vi "test_EnumerateServicesWrapper_RunEnumerateServices_ReturnsAvailableServices.vi"(8 "error in":errorcluster) -> (0 "error out":errorcluster, 2 "result":string, 3 "pass":bool)   [LabVIEW 2021, in "MeasurementServerTests.lvlib" / "Discovery Tests.lvlib"]
uses:
  Discovery Tests.lvlib
  MeasurementServerTests.lvlib
  gRPC/Generated APIs/ni/measurementlink/discovery/v1/RPC Messages/ni_measurementlink_discovery_v1_EnumerateServicesRequest.ctl
  gRPC/Generated APIs/ni/measurementlink/discovery/v1/ni.measurementlink.discovery.v1.api.lvlib
  Runtime/Clients/Discovery V1/NI Discovery V1 Client.lvlib
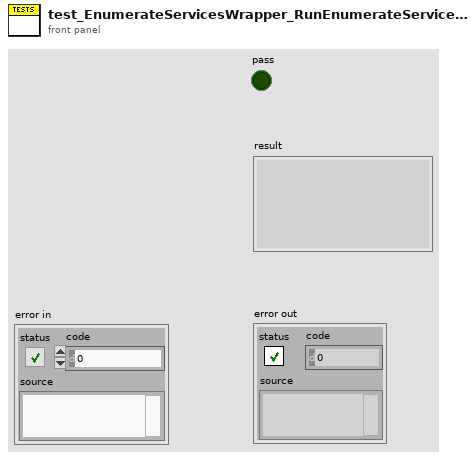
[diagram p1: front panel]
types:
  T1 = typedef "ni.measurementlink.discovery.v1.api.lvlib/ni_measurementlink_discovery_v1_EnumerateServicesRequest.ctl" = cluster{"provided_interface":string}
  T2 = typedef "ni.measurementlink.discovery.v1.api.lvlib/ni_measurementlink_discovery_v1_EnumerateServicesResponse.ctl" = cluster{"available_services":T3[]}
  T3 = typedef "ni.measurementlink.discovery.v1.api.lvlib/ni_measurementlink_discovery_v1_ServiceDescriptor.ctl" = cluster{"display_name":string, "description_url":string, "provided_interfaces":string[], "service_class":string, "annotations":T4[]}
  T4 = typedef "ni.measurementlink.discovery.v1.api.lvlib/ni_measurementlink_discovery_v1_ServiceDescriptor_AnnotationsEntry.ctl" = cluster{"key":string, "value":string}
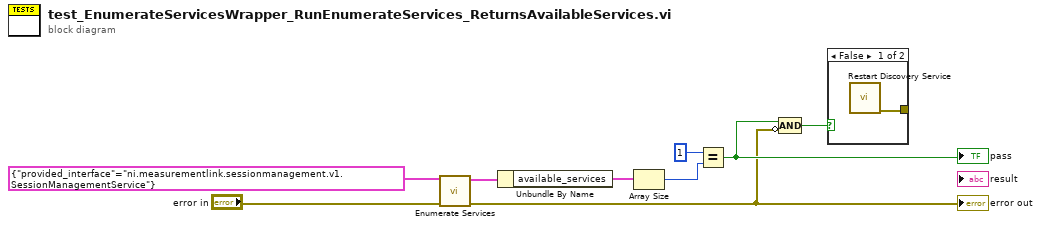
[diagram p0: block diagram]
diagram:
  n1 = call "Enumerate Services.vi"("error in"="error in", "request data"=T1 {"provided_interface"="ni.measurementlink.sessionmanagement.v1.SessionManagementService"}) -> ("error out"=w3:errorcluster, "response data"=w1:T2)  [unwired: 7 in]
  "error out" <- w3
  n2 = Unbundle By Name(w1) -> ("available_services"=w7:T3[])
  n3 = Array Size(array=w7) -> (size(s)=w6:i32)
  n4 = Equal?(x=1, y=w6) -> (x = y?=w4:bool)
  "pass" <- w4
  n5 = Compound Arithmetic op=AND(w4, invert w3) -> (w8:bool)
  n6 = case shown="False" w8 {
    tunnel: [w10 _] -> _
    frame False {
      n7 = call "Restart Discovery Service.vi"() -> ("error out"=w10:errorcluster)  [unwired: 11 in]
    }
    frame True {
    }
  }
